vi "CleanUpBeats.vi"(11 "Beat INput":dbl[][](array[numeric])=[[121.51943772061755, 420.00118010440303, 737.3356624901787, 0.0, 0.0, 0.0], [205.82219676408096, 493.31698893022036, 815.9428102570546, 0.0, 0.0, 0.0], [299.7453935518194, 597.9648550021464, 934.04011517869, 0.0, 0.0, 0.0], [88.4078085074326, 395.1698392203118, 716.8190090287251, 0.0, 0.0, 0.0], [244.1857740016493, 550.4869993758543, 856.1700414331177, 0.0, 0.0, 0.0], [33.32933013344357, 324.00409479181104, 631.5204898608247, 973.3220169387411, 0.0, 0.0], [105.67386629498925, 427.47499380582815, 722.9782752736321, 0.0, 0.0, 0.0], [189.9812681292953, 492.96169685404544, 817.0591843623589, 0.0, 0.0, 0.0], [228.199227736101, 525.6638231002262, 857.6044825201323, 0.0, 0.0, 0.0], [58.23889160918931, 403.22555237489473, 688.2505747467349, 0.0, 0.0, 0.0], [225.17689140667437, 532.1057034333368, 848.9167710099598, 0.0, 0.0, 0.0], [36.296023531566824, 344.3892176106879, 642.8075193093929, 965.8075238817241, 0.0, 0.0], [121.10113270980241, 441.68544771176005, 752.695991450584, 0.0, 0.0, 0.0], [251.48774428681114, 572.4791630543307, 869.176690878975, 0.0, 0.0, 0.0], [52.46873359035273, 395.47504062591366, 674.9865637552624, 972.1270682506312, 0.0, 0.0], [244.02011394065278, 531.4284066999393, 852.307491100627, 0.0, 0.0, 0.0], [72.4399324521319, 389.6742427791761, 693.5311968251567, 0.0, 0.0, 0.0], [246.37076591338464, 882.2648235920902, 0.0, 0.0, 0.0, 0.0], [217.11028766167126, 520.7361118187919, 835.3786814721568, 0.0, 0.0, 0.0], [426.43223139541516, 763.9570983443334, 0.0, 0.0, 0.0, 0.0], [80.91976182094804, 424.8182953368139, 719.3362552599889, 0.0, 0.0, 0.0], [114.34581735580875, 271.2127951043793, 618.0954839620413, 926.1094361181123, 0.0, 0.0], [26.246848829810478, 300.2966678431457, 627.1657000232011, 947.4044800627787, 0.0, 0.0], [256.38650360221436, 908.3233895096832, 0.0, 0.0, 0.0, 0.0], [404.9071630337426, 0.0, 0.0, 0.0, 0.0, 0.0], [155.44963005829123, 480.0080837791027, 832.2125063066728, 958.1767038426171, 0.0, 0.0], [55.50271148381487, 394.5137053737926, 528.3739815820318, 689.2316021611833, 0.0, 0.0], [112.90803311481335, 447.4545009777395, 740.7478007581221, 0.0, 0.0, 0.0], [39.78481411488089, 218.51049054536088, 265.7335847824247, 413.6101959802887, 670.9612209505653, 972.7287416066438], [96.20374578033767, 404.414936834101, 630.0163278422308, 800.3941924987346, 924.7486300123105, 0.0], [179.35946895479736, 502.05898793046276, 708.210368857032, 864.3680944967618, 0.0, 0.0], [169.30625128437634, 222.76132584764255, 595.6718013460664, 717.2274234980033, 939.3100901495663, 0.0], [27.919263602700767, 191.428317757865, 307.5803058983347, 540.2053681592004, 652.0283786534758, 961.8222455096045], [32.34350393250323, 358.33487551738904, 659.3463401316069, 970.8009773355457, 0.0, 0.0], [192.8434387004087, 515.0037529557882, 839.1610480439731, 0.0, 0.0, 0.0], [64.22436502029983, 389.38431632573685, 703.063139273003, 0.0, 0.0, 0.0], [184.24328316758127, 489.3687671968337, 616.7519587372843, 0.0, 0.0, 0.0], [242.0040045745327, 582.1414992065841, 918.0457114278594, 0.0, 0.0, 0.0], [220.68720142586804, 584.5676493769168, 889.8662621577093, 0.0, 0.0, 0.0], [220.83519577969116, 544.0362248908528, 914.102031523041, 0.0, 0.0, 0.0], [242.2253545141312, 563.6821139881953, 914.8949021551127, 0.0, 0.0, 0.0], [31.36764210747541, 640.624814396431, 967.2586478034925, 0.0, 0.0, 0.0], [26.118026704047836, 286.52148719178575, 627.3241409267392, 0.0, 0.0, 0.0], [199.31092011080676, 537.6134776299749, 881.4270202470025, 0.0, 0.0, 0.0], [241.44193381081766, 575.4192366160279, 0.0, 0.0, 0.0, 0.0], [221.06957863163956, 532.4521130365349, 0.0, 0.0, 0.0, 0.0], [159.68133103967455, 477.1865189343335, 0.0, 0.0, 0.0, 0.0], [101.07021610324765, 426.5690827698043, 733.9737359426038, 0.0, 0.0, 0.0], [83.93330793359097, 433.93515078091036, 718.506175318371, 0.0, 0.0, 0.0], [39.653439981083224, 679.3157837414819, 974.1726144597444, 0.0, 0.0, 0.0], [277.8756012316641, 614.7819690105323, 0.0, 0.0, 0.0, 0.0], [195.79296030579593, 516.054454407788, 830.1947965810825, 0.0, 0.0, 0.0], [84.05615068582145, 424.92646415574393, 718.0366722217861, 0.0, 0.0, 0.0], [176.02585355417082, 513.672543559361, 819.6683640653889, 0.0, 0.0, 0.0], [191.22198928675363, 523.5507006324474, 815.3792588159404, 0.0, 0.0, 0.0], [136.64496852405193, 479.3411658343035, 781.2355267240156, 0.0, 0.0, 0.0], [87.03493782361565, 703.0537470934951, 0.0, 0.0, 0.0, 0.0], [50.26624628655964, 692.1421178651668, 0.0, 0.0, 0.0, 0.0], [55.56167375673223, 672.8269764413058, 0.0, 0.0, 0.0, 0.0], [113.32015158034643, 473.7018131297216, 733.5593449160226, 0.0, 0.0, 0.0], [165.83260199187106, 484.2576579138015, 785.9861400985046, 0.0, 0.0, 0.0], [279.9668878111462, 610.614102162891, 962.970516629822, 0.0, 0.0, 0.0], [158.55471363005407, 463.72800596010285, 778.8629287653853, 0.0, 0.0, 0.0], [97.50923625372889, 445.66760025772896, 744.2307691439161, 0.0, 0.0, 0.0], [275.00530284019135, 601.3092946159268, 961.2920759404703, 0.0, 0.0, 0.0], [106.20868062457117, 441.5722422712855, 734.9878848308458, 0.0, 0.0, 0.0], [250.76492485627583, 574.0208586253901, 0.0, 0.0, 0.0, 0.0], [83.89594572520669, 439.4924917813438, 712.672057649843, 0.0, 0.0, 0.0], [209.1982390151692, 515.2769706741772, 830.7023456136573, 0.0, 0.0, 0.0], [30.34457448941511, 321.7201013709873, 625.6902776902057, 0.0, 0.0, 0.0], [104.1576519697571, 443.3799664807947, 755.9982676801217, 0.0, 0.0, 0.0], [216.64093505056977, 541.829614817203, 848.2250873010589, 0.0, 0.0, 0.0], [280.1608129300152, 614.3218659821921, 958.498486876028, 0.0, 0.0, 0.0], [109.53251907747219, 449.7637930466675, 737.5983486252154, 0.0, 0.0, 0.0], [257.07079718690585, 600.6382288986334, 944.2335933020586, 0.0, 0.0, 0.0], [193.65785650394406, 502.6907044840901, 811.9019581314631, 0.0, 0.0, 0.0], [86.71439551469878, 424.00603941809266, 694.774010161043, 0.0, 0.0, 0.0], [240.60062801945168, 541.5566628077322, 0.0, 0.0, 0.0, 0.0], [165.82532095758046, 500.14873398322777, 0.0, 0.0, 0.0, 0.0], [134.4735428193173, 443.49326121691865, 756.0051479523423, 0.0, 0.0, 0.0], [55.76549292114746, 413.4115571494036, 687.0100043637832, 0.0, 0.0, 0.0], [280.17530780041085, 591.6005814604266, 938.8297765075215, 0.0, 0.0, 0.0], [165.5375050356032, 487.6300183122374, 801.0306859483433, 0.0, 0.0, 0.0], [73.34487283162593, 414.5082602632136, 689.8599719649185, 0.0, 0.0, 0.0], [276.01522100203096, 587.006002390357, 944.481385032788, 0.0, 0.0, 0.0], [135.2225706059279, 466.48133447386476, 764.3789622646332, 0.0, 0.0, 0.0], [32.988836001112745, 650.9885742666509, 0.0, 0.0, 0.0, 0.0], [203.28603636603327, 512.5961518144832, 0.0, 0.0, 0.0, 0.0], [67.75846467618413, 702.8641801872328, 0.0, 0.0, 0.0, 0.0], [262.8730113198678, 567.427151041079, 946.0051589301988, 0.0, 0.0, 0.0], [135.57073090427107, 447.82811357303547, 749.1439479960125, 0.0, 0.0, 0.0], [114.49028234201427, 448.85737964375573, 759.7001938634189, 0.0, 0.0, 0.0], [31.63804815681346, 656.0238172878908, 972.0448040373165, 0.0, 0.0, 0.0], [211.09452230850076, 513.6961671634378, 814.6149347768933, 0.0, 0.0, 0.0], [89.16121034320719, 422.4102121917276, 713.4562067405056, 0.0, 0.0, 0.0], [56.11501416489475, 410.8546406137114, 697.1106555092862, 0.0, 0.0, 0.0], [273.79727262987956, 577.2940596981827, 942.4302231679419, 0.0, 0.0, 0.0], [127.21674155515923, 441.69298786115934, 764.5307584177199, 0.0, 0.0, 0.0], [36.83102101965137, 370.3269731755343, 654.6501938730387, 958.5264375619674, 0.0, 0.0], [29.456189466984075, 304.33712086767605, 632.5913059066406, 954.0776574157933, 0.0, 0.0], [259.9052814107479, 608.0004359112426, 935.4528390057645, 0.0, 0.0, 0.0], [216.38622176110243, 530.7325098290642, 891.9128698129576, 0.0, 0.0, 0.0], [192.30346505486165, 510.5487352833404, 855.9536293273641, 0.0, 0.0, 0.0], [253.12718521602403, 562.5106335730807, 920.9025262188845, 0.0, 0.0, 0.0], [150.50171824153995, 470.25825929492413, 768.5340237253249, 0.0, 0.0, 0.0], [211.97147803588103, 521.6942142382136, 850.6164249879541, 0.0, 0.0, 0.0], [146.2330298772437, 453.8743209374667, 778.2933820845797, 0.0, 0.0, 0.0], [129.1060065168295, 442.6674745798166, 799.5853599367899, 0.0, 0.0, 0.0], [83.22074568625195, 395.8818115070186, 708.1115662464556, 0.0, 0.0, 0.0], [148.2805404429883, 453.4797210473197, 778.7729245414745, 0.0, 0.0, 0.0], [159.33675528020808, 456.2624278394679, 785.250215196356, 0.0, 0.0, 0.0], [111.51040792662033, 445.6635584535485, 748.6519855067013, 0.0, 0.0, 0.0], [384.47265630762854, 729.8854116645057, 0.0, 0.0, 0.0, 0.0], [279.14942330239415, 627.6838829298432, 935.9219646239032, 0.0, 0.0, 0.0], [244.0257391859101, 552.1490907571929, 858.8028894915592, 0.0, 0.0, 0.0], [92.2789498338786, 431.0413877754123, 724.7046701406098, 0.0, 0.0, 0.0], [78.96363190642207, 414.79025405476824, 718.8681959487624, 0.0, 0.0, 0.0], [96.87654944062015, 408.8598039596226, 722.1286682042411, 0.0, 0.0, 0.0], [46.78748516735247, 405.1286242113334, 683.0886323900238, 0.0, 0.0, 0.0], [149.10467048670955, 461.74478845199496, 794.9732124625926, 0.0, 0.0, 0.0], [199.6701997158832, 505.4497220244601, 865.1711815737027, 0.0, 0.0, 0.0], [265.44333105298097, 591.2557083184657, 913.4568479496622, 0.0, 0.0, 0.0], [44.006234218924405, 399.6623155002208, 681.3342486308367, 973.8521209475576, 0.0, 0.0], [49.99473377161078, 400.4431586113403, 683.3809368494226, 0.0, 0.0, 0.0], [32.705789974256106, 300.05229796692765, 627.868752603526, 969.5725133500232, 0.0, 0.0], [160.4205949757276, 474.48391214695914, 781.2033689927439, 0.0, 0.0, 0.0], [27.833361060743588, 308.50159179667327, 649.611463696074, 0.0, 0.0, 0.0], [81.53491407874367, 426.4638795906131, 720.7066074279378, 0.0, 0.0, 0.0], [238.1530397553242, 563.5299089424241, 853.1609772973668, 0.0, 0.0, 0.0], [29.88716167501594, 302.76399091354585, 634.1976503619833, 973.1810663242369, 0.0, 0.0], [109.38094610067891, 461.38697455752765, 754.6786753894887, 0.0, 0.0, 0.0], [153.00713499365594, 495.3808009590821, 800.0443236471953, 0.0, 0.0, 0.0], [97.95555778603622, 728.6980906176937, 0.0, 0.0, 0.0, 0.0], [48.42564286126757, 352.86604000069957, 681.713537501161, 0.0, 0.0, 0.0], [27.57719340744371, 332.19160605388913, 632.4011898422343, 944.7349602507185, 0.0, 0.0], [229.0708893518776, 530.1471031122553, 852.2214568662881, 0.0, 0.0, 0.0], [175.68330972081768, 483.3134870562433, 844.6243505059398, 0.0, 0.0, 0.0], [172.64958480619242, 492.8478358699961, 802.4662657865397, 0.0, 0.0, 0.0], [158.86853288376864, 478.7345421549702, 792.0252891791572, 0.0, 0.0, 0.0], [108.23784678769, 447.2855276076152, 772.7185168674448, 0.0, 0.0, 0.0], [27.381694915128627, 294.1193040353853, 628.1181847847432, 973.6498319296936, 0.0, 0.0], [516.702015549951, 826.5444650434202, 0.0, 0.0, 0.0, 0.0], [46.08262810333208, 414.87354495618035, 697.4820290480967, 0.0, 0.0, 0.0], [210.97484365776955, 526.1310619987623, 841.7286570165653, 0.0, 0.0, 0.0], [42.221500236297075, 377.6467053635791, 671.6087962940703, 0.0, 0.0, 0.0], [164.14151634830176, 466.2303441610503, 787.5565178670483, 0.0, 0.0, 0.0], [84.85605825546912, 428.3928285467387, 723.5089416204362, 0.0, 0.0, 0.0], [192.11327254689718, 500.96461340084016, 828.8772823733012, 0.0, 0.0, 0.0], [279.78612579527464, 610.3856657625397, 0.0, 0.0, 0.0, 0.0], [125.17278186903766, 434.5919896084132, 759.0077716811652, 0.0, 0.0, 0.0], [78.32707708209132, 390.33071538355335, 695.7972828779745, 0.0, 0.0, 0.0], [44.922247432446184, 407.01280184728313, 698.2052586209891, 0.0, 0.0, 0.0], [190.2857243913234, 497.68739030486665, 833.402545220205, 0.0, 0.0, 0.0], [428.73032340159494, 745.8634779244865, 0.0, 0.0, 0.0, 0.0], [31.456918770399483, 334.90633992166397, 674.8068959273003, 969.3020149956751, 0.0, 0.0], [211.889253358806, 531.622094766208, 855.0235763592015, 0.0, 0.0, 0.0], [38.724653742014084, 333.70697145228803, 681.514271065534, 0.0, 0.0, 0.0], [198.88771017424529, 518.829973274344, 853.584577906026, 0.0, 0.0, 0.0], [45.117456461491614, 403.07244611787274, 683.8200967709652, 0.0, 0.0, 0.0], [248.24918971319292, 557.7473153092069, 896.2746755393084, 0.0, 0.0, 0.0], [129.64579854106705, 434.07009702560504, 769.5078929709325, 0.0, 0.0, 0.0], [292.29883953996057, 613.916081240957, 957.7896035054001, 0.0, 0.0, 0.0], [154.6716708457954, 479.9242170984537, 792.4351802534841, 0.0, 0.0, 0.0], [143.22683259848665, 474.24675027671316, 779.6158448489001, 0.0, 0.0, 0.0], [34.15040720426349, 356.3360689196114, 967.7778436743794, 0.0, 0.0, 0.0], [256.7767128482131, 576.0738595872083, 956.660870803041, 0.0, 0.0, 0.0], [158.62878143937252, 472.23928604503965, 831.4545215624514, 0.0, 0.0, 0.0], [81.3922758342585, 395.18103752455386, 744.0690009214122, 0.0, 0.0, 0.0], [103.81120627272742, 440.9195635556064, 731.9246794721446, 0.0, 0.0, 0.0], [63.25140112914518, 399.5389673306159, 0.0, 0.0, 0.0, 0.0], [31.74043273335791, 344.2003886622516, 661.3474673657815, 961.3661082655021, 0.0, 0.0], [55.70317566712425, 428.75132357239954, 726.3861344068887, 0.0, 0.0, 0.0], [130.61469013611344, 441.1530516147307, 789.4089075574203, 0.0, 0.0, 0.0], [220.57699722401298, 561.9888534769188, 890.7568668215732, 0.0, 0.0, 0.0], [27.573721466455684, 363.3959683969656, 654.1802773982168, 947.7056736828706, 0.0, 0.0], [32.23747112640801, 369.84271983521944, 671.1998290808133, 968.8115841386852, 0.0, 0.0], [72.29801010653493, 381.32244252823523, 724.0372620921694, 0.0, 0.0, 0.0], [160.83934695494824, 475.204355648481, 830.3258393743622, 0.0, 0.0, 0.0], [140.73221290333913, 773.3603460057811, 0.0, 0.0, 0.0, 0.0], [281.7235121234386, 625.5499268800227, 973.295929229484, 0.0, 0.0, 0.0], [146.1293690173475, 456.2801406653385, 0.0, 0.0, 0.0, 0.0]]) -> (2 "final mean":dbl format="%0.2f", 3 "Beat Ref Marks":dbl[][](array[numeric]))   [LabVIEW 2022 SP3]
uses:
  <vilib>/Analysis/baseanly.llb/Mean (DBL).vi
  <vilib>/Analysis/NI_AALBase.lvlib
panel:
  out "Splits 2":dbl[][](array[numeric])
  out "Splits":dbl[][](array[numeric])
  out "Array":dbl[](array[numeric])
  out "Start Mean":dbl format="%0.2f"
  out "Start Differences":dbl[](graph)
  out "Final Differences":dbl[](graph)
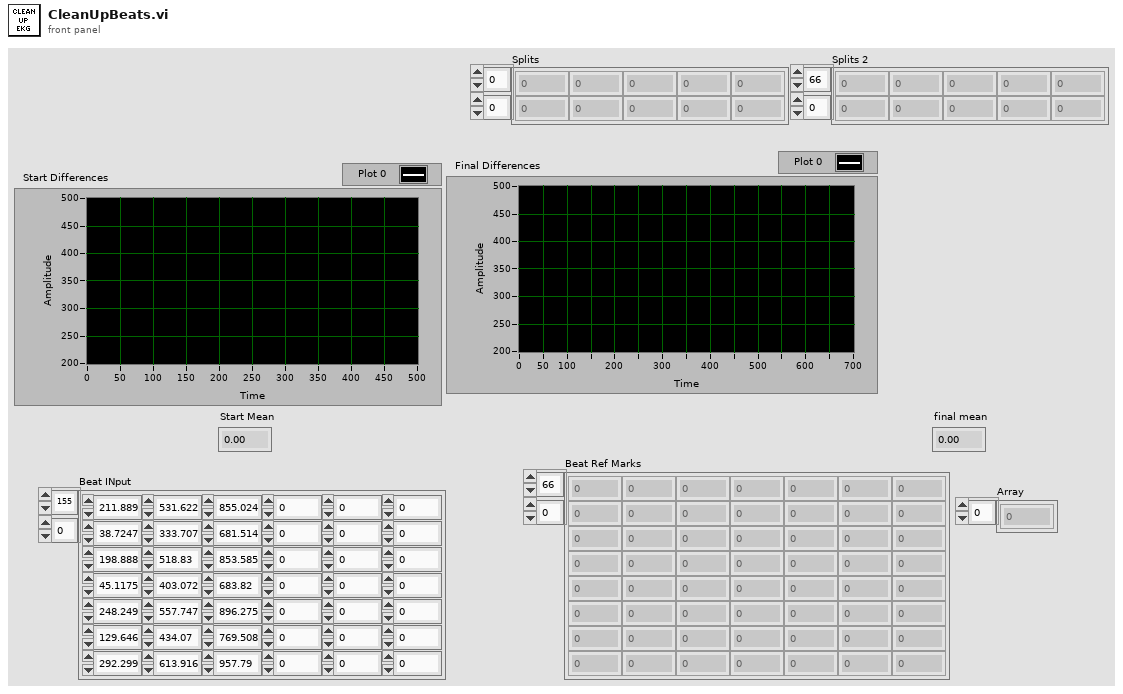
[diagram p1: front panel]
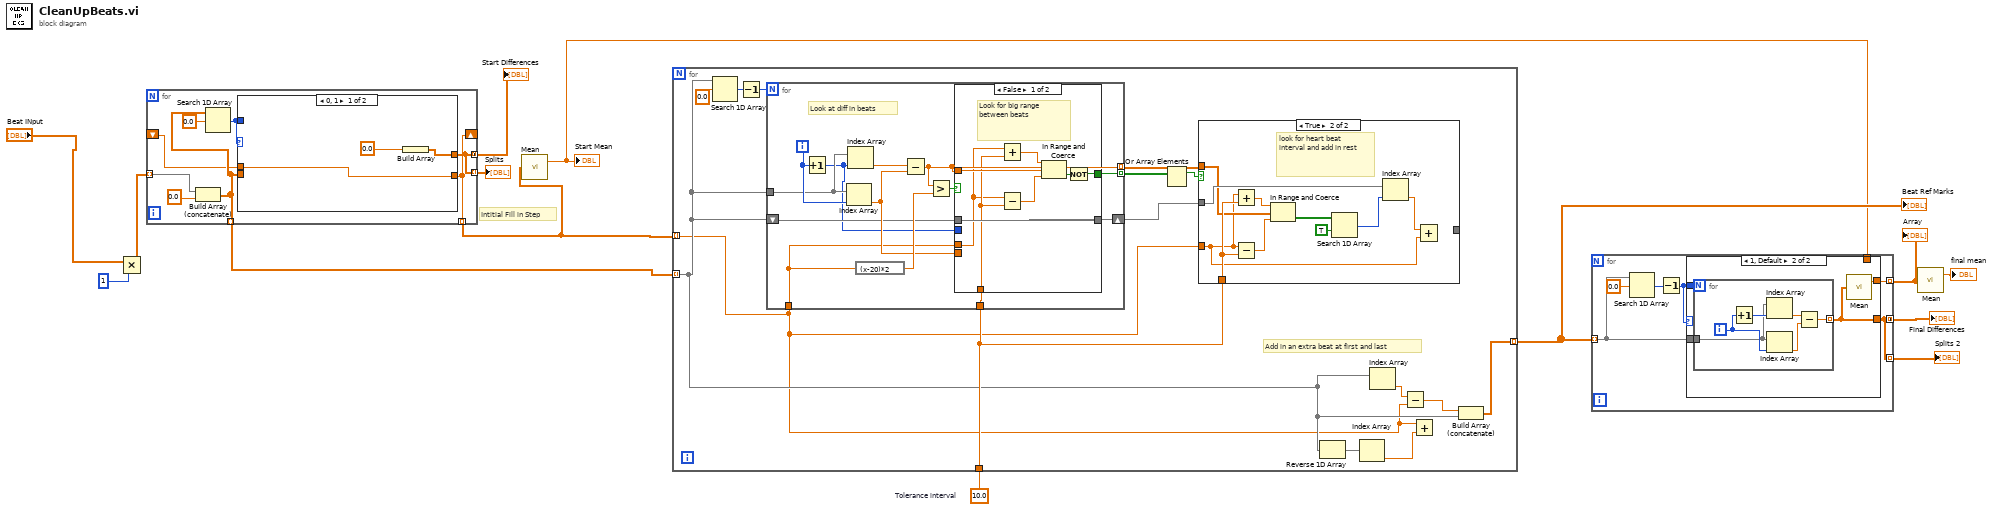
[diagram p0: block diagram]
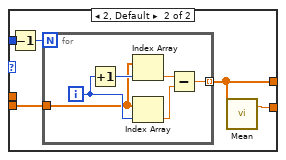
[diagram p2: hidden frame]
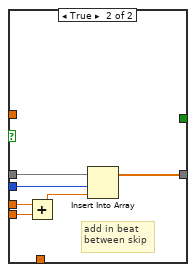
[diagram p5: hidden frame]
diagram:
  w12 = 10.0  # Tolerance interval
  # "Intitial Fill in Step"
  n1 = Multiply(x="Beat INput", y=1) -> (x*y=w5:dbl[][])
  n2 = for {
    tunnel: w5 -> [w20] mode=indexing
    tunnel: [w15] -> w11 mode=concatenating
    tunnel: [w18] -> w10 mode=indexing
    tunnel: [w19] -> w7 mode=indexing
    shift-right: [w18] -> _
    shift-left: _ -> [w17]
    tunnel: [w15] -> w3 mode=indexing
    n3 = Build Array (concatenate)(w20, 0.0) -> (w19:dbl[])
    n4 = Search 1D Array(1D array=w19, element=0.0) -> (index of element=w16:i32)  [unwired: 1 in]
    n5 = case shown="0, 1" w16 {
      tunnel: w16 -> [_ w29]
      tunnel: [w24 w28] -> w15
      tunnel: w19 -> [_ w27]
      tunnel: [w25 w26] -> w18
      tunnel: w17 -> [w25 _]
      frame 0, 1 {
        n6 = Build Array(0.0 ("element")) -> (w24:dbl[])
      }
      frame 2, Default {
        n7 = Decrement(x=w29) -> (x-1=w30:i32)
        n8 = for {
          N: w30 -> [_]
          tunnel: [w34] -> w28 mode=indexing
          tunnel: w27 -> [w31]
          i -> [w33]
          n9 = Increment(x=w33) -> (x+1=w36:i32)
          n10 = Index Array(array=w31, index=w36) -> (element=w35:dbl)
          n11 = Index Array(array=w31, index=w33) -> (element=w32:dbl)
          n12 = Subtract(x=w35, y=w32) -> (x-y=w34:dbl)
        }
        n13 = call-poly <vilib>:"Mean.vi"("X"=w28) -> ("mean"=w26:dbl)  [unwired: 1 out]
      }
    }
  }
  "Start Differences" <- w11
  "Splits" <- w3
  n14 = call-poly <vilib>:"Mean.vi"("X"=w10) -> ("mean"=w4:dbl)  [unwired: 1 out]
  "Start Mean" <- w4
  n15 = for {
    tunnel: w7 -> [w39] mode=indexing
    tunnel: [w37] -> w13 mode=indexing
    tunnel: w12 -> [w40]
    tunnel: w10 -> [w38] mode=indexing
    # "Add in an extra beat at first and last"
    n16 = Search 1D Array(1D array=w39, element=0.0) -> (index of element=w50:i32)  [unwired: 1 in]
    n17 = Decrement(x=w50) -> (x-1=w51:i32)
    n18 = for {
      N: w51 -> [_]
      tunnel: [w66] -> w45 mode=indexing
      tunnel: w38 -> [w64]
      shift-right: [w70] -> w46
      shift-left: w39 -> [w68]
      tunnel: w39 -> [w69]
      tunnel: [w65] -> w48 mode=indexing
      tunnel: w40 -> [w63]
      i -> [w72]
      # "Look at diff in beats"
      n19 = Increment(x=w72) -> (x+1=w67:i32)
      n20 = Index Array(array=w69, index=w72) -> (element=w71:dbl)
      n21 = Index Array(array=w69, index=w67) -> (element=w75:dbl)
      n22 = expression code="(x-20)*2"(w64) -> (w74:dbl)
      n23 = Subtract(x=w75, y=w71) -> (x-y=w66:dbl)
      n24 = Greater?(x=w66, y=w74) -> (0:w73:bool)
      n25 = case shown="False" w73 {
        tunnel: w68 -> [w83 w89]
        tunnel: w67 -> [_ w88]
        tunnel: w64 -> [w76 w87]
        tunnel: w71 -> [_ w86]
        tunnel: [w83 w84] -> w70
        tunnel: w66 -> [w79 _]
        tunnel: [w78 _] -> w65
        tunnel: w63 -> [w77 _]
        frame False {
          # "Look for big range between beats"
          n26 = Add(x=w76, y=w77) -> (x+y=w82:dbl)
          n27 = Subtract(x=w76, y=w77) -> (x-y=w81:dbl)
          n28 = In Range and Coerce(upper limit=w82, x=w79, lower limit=w81) -> (In Range?=w80:bool)  [unwired: 1 out]
          n29 = Not(x=w80) -> (.not. x?=w78:bool)
        }
        frame True {
          # "add in beat \nbetween skip"
          n30 = Add(x=w87, y=w86) -> (x+y=w85:dbl)
          n31 = Insert Into Array(array=w89, index=w88, new element=w85) -> (w84:dbl[])
        }
      }
    }
    n32 = Or Array Elements(Boolean array=w48) -> (logical OR=w47:bool)
    n33 = case shown="True" w47 {
      tunnel: w46 -> [w52 w58]
      tunnel: [w52 _] -> _
      tunnel: w38 -> [_ w53]
      tunnel: w45 -> [_ w54]
      tunnel: w40 -> [_ w55]
      frame False {
      }
      frame True {
        # "look for heart beat interval and add in rest"
        n34 = Add(x=w53, y=w55) -> (x+y=w62:dbl)
        n35 = Subtract(x=w53, y=w55) -> (x-y=w61:dbl)
        n36 = In Range and Coerce(upper limit=w62, x=w54, lower limit=w61) -> (In Range?=w60:bool[])  [unwired: 1 out]
        n37 = Search 1D Array(1D array=w60, element=TRUE) -> (index of element=w57:i32)  [unwired: 1 in]
        n38 = Index Array(array=w58, index=w57) -> (element=w56:dbl)
        n39 = Add(x=w56, y=w53) -> ()  [unwired: 1 out]
      }
    }
    n40 = Reverse 1D Array(array=w39) -> (reversed array=w42:dbl[])
    n41 = Index Array(array=w42) -> (element=w41:dbl)  [unwired: 1 in]
    n42 = Index Array(array=w39) -> (element=w44:dbl)  [unwired: 1 in]
    n43 = Subtract(x=w44, y=w38) -> (x-y=w43:dbl)
    n44 = Add(x=w38, y=w41) -> ()  [unwired: 1 out]
    n45 = Build Array (concatenate)(w43, w39) -> (w37:dbl[])
  }
  "Beat Ref Marks" <- w13
  n46 = for {
    tunnel: w13 -> [w94] mode=indexing
    tunnel: [w90] -> w14 mode=concatenating
    tunnel: [w93] -> w9 mode=indexing
    tunnel: w4 -> [w91]
    tunnel: [w90] -> w2 mode=indexing
    n47 = Search 1D Array(1D array=w94, element=0.0) -> (index of element=w96:i32)  [unwired: 1 in]
    n48 = Decrement(x=w96) -> (x-1=w92:i32)
    n49 = case shown="1, Default" w92 {
      tunnel: w92 -> [_ w101]
      tunnel: w94 -> [_ w100]
      tunnel: [_ w99] -> w90
      tunnel: [w97 w98] -> w93
      tunnel: w91 -> [w97 _]
      frame -1, 0 {
      }
      frame 1, Default {
        n50 = for {
          N: w101 -> [_]
          tunnel: [w105] -> w99 mode=indexing
          tunnel: w100 -> [w102]
          i -> [w104]
          n51 = Increment(x=w104) -> (x+1=w107:i32)
          n52 = Index Array(array=w102, index=w107) -> (element=w106:dbl)
          n53 = Index Array(array=w102, index=w104) -> (element=w103:dbl)
          n54 = Subtract(x=w106, y=w103) -> (x-y=w105:dbl)
        }
        n55 = call-poly <vilib>:"Mean.vi"("X"=w99) -> ("mean"=w98:dbl)  [unwired: 1 out]
      }
    }
  }
  "Final Differences" <- w14
  "Array" <- w9
  "Splits 2" <- w2
  n56 = call-poly <vilib>:"Mean.vi"("X"=w9) -> ("mean"=→"final mean":dbl)  [unwired: 1 out]
